vi "Get Plugins.vi"(8 "error in (no error)":errorcluster, 11 "Framework Ref in":T1 format="%.0x") -> (0 "error out":errorcluster, 2 "Plugin refs":T1[](array[typedef]) format="%.0x", 3 "Framework Ref out":T1 format="%.0x")   [LabVIEW 2017, in "DSF Shared.lvlib"]
uses:
  Shared/DSF Shared.lvlib
  <vilib>/NI Veristand/Custom Device API/Custom Device Item Ref.ctl
  Shared/Plugin Page GUID.vi
  <vilib>/NI Veristand/Custom Device API/Custom Device API.lvlib
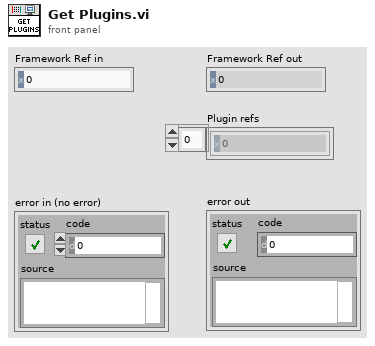
[diagram p1: front panel]
types:
  T1 = typedef "Custom Device API.lvlib/Custom Device Item Ref.ctl" = u64
  T2 = typedef "Custom Device API.lvlib/Custom Device Item Info.ctl" = cluster{"Name":string, "Is Channel":bool, "GUID":string, "Is Waveform":bool}
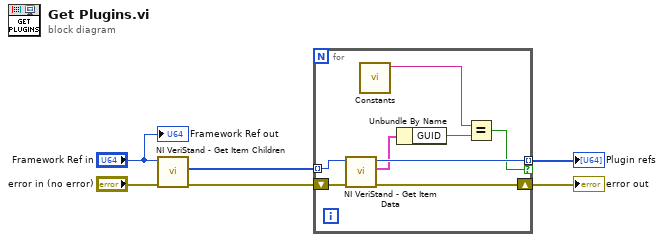
[diagram p0: block diagram]
diagram:
  n1 = call <vilib>:"NI VeriStand - Get Item Children.vi"("error in (no error)"="error in (no error)", "Item Ref in"="Framework Ref in") -> ("error out"=w5:errorcluster, "Child Refs"=w3:T1[])  [unwired: 6 in, 2 out]
  n2 = for {
    shift-right: [w13] -> w2
    shift-left: w5 -> [w14]
    tunnel: w3 -> [w12] mode=indexing
    tunnel: [w9] -> w1 mode=indexing if=w8
    n3 = call <vilib>:"NI VeriStand - Get Item Data.vi"("error in (no error)"=w14, "Item Ref in"=w12) -> ("error out"=w13:errorcluster, "Item Info"=w7:T2, "Item Ref out"=w9:T1)  [unwired: 6 in, 1 out]
    n4 = call-poly "Constants.vi"() -> ("Plugin GUID"=w11:string)  [unwired: 11 in]
    n5 = Unbundle By Name(w7) -> ("GUID"=w10:string)
    n6 = Equal?(x=w11, y=w10) -> (x = y?=w8:bool)
  }
  "error out" <- w2
  "Plugin refs" <- w1
  "Framework Ref out" <- "Framework Ref in"
